vi "Format Basic Bullet List.vi"(8 "Error in":errorcluster caption="Error in (no error)", 11 "String Array":string[](array[string])) -> (0 "Error out":errorcluster, 3 "Bullet List":string)   [LabVIEW 2023, in "Confluence Formatting.lvlib"]
uses:
  Confluence Formatting.lvlib
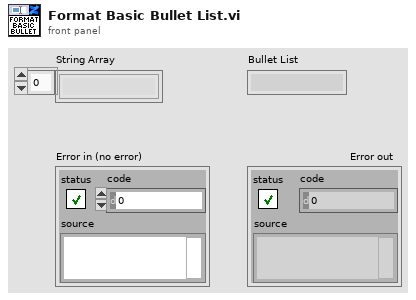
[diagram p1: front panel]
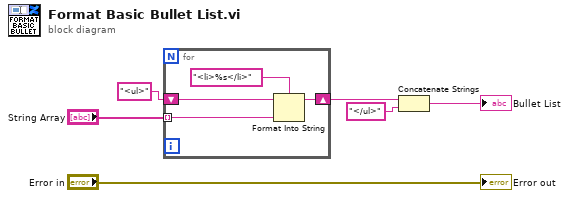
[diagram p0: block diagram]
diagram:
  n1 = for {
    shift-right: [w7] -> w3
    shift-left: "<ul>" -> [w10]
    tunnel: "String Array" -> [w8] mode=indexing
    n2 = Format Into String(format string="<li>%s</li>", initial string=w10, w8) -> (resulting string=w7:string)  [unwired: 1 in, 1 out]
  }
  n3 = Concatenate Strings(w3, "</ul>" ("string")) -> (→"Bullet List":string)
  "Error out" <- "Error in"
